vi "FPGA_lock-in_generat-light.vi"() -> ()   [LabVIEW 2010]
uses:
  fast cycles/FPGA_run-states.ctl
  <vilib>/rvi/DataTransferAndStorage/Container/XNode/niFpgaContainer.xnode
  <vilib>/eio/EIONode/EIONode.xnode
  <vilib>/rvi/eio/nirviEIOImplementation/nirviEIOImplementation.xnode
  <vilib>/rvi/eio/common/nirviEmuClasses.ctl
  <vilib>/rvi/FIFO/Fifo_Resource/nirvififoEmulationSetSize.vi
  <vilib>/rvi/DataTransferAndStorage/Container/Common/niFpgaContainerGetUniqueNameForEmu.vi
  <vilib>/rvi/Memory/Memory_Emulation/nirvimemoryEmulationManagerCache_GetValue.vi
  <vilib>/rvi/Memory/Memory_Emulation/nirvimemoryEmulationManagerCache_InsertValue.vi
  <vilib>/Utility/error.llb/Clear Errors.vi
  <vilib>/rvi/Memory/Memory_Emulation/nirvimemoryEmulationManagerCache_SetValue.vi
  <vilib>/rvi/eio/common/nirviEmuTemplateMethod_noerrors.vi
panel:
  in  "DAC mem adr":u8
  out "LI channel":u16
  in  "inhibate lock-in":bool=TRUE
  in  "clock reset":bool
  in  "clock divider":u32=20
  in  "Amplitude":fxp<+/-,16,16>
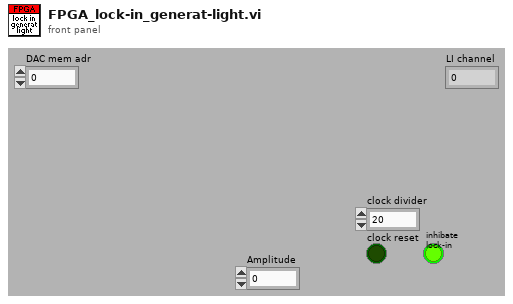
[diagram p1: front panel]
types:
  T1 = typedef "FPGA_run-states.ctl" = enum16{"stopped", "check", "reserve", "run", "release"}
  T2 = cluster{"Boolean array[0]":bool, "Boolean array[1]":bool}
  T3 = typedef "nirviEmuClasses.ctl" = enum16{"IO Read", "IO Write", "Method", "Property Read", "Property Write"}
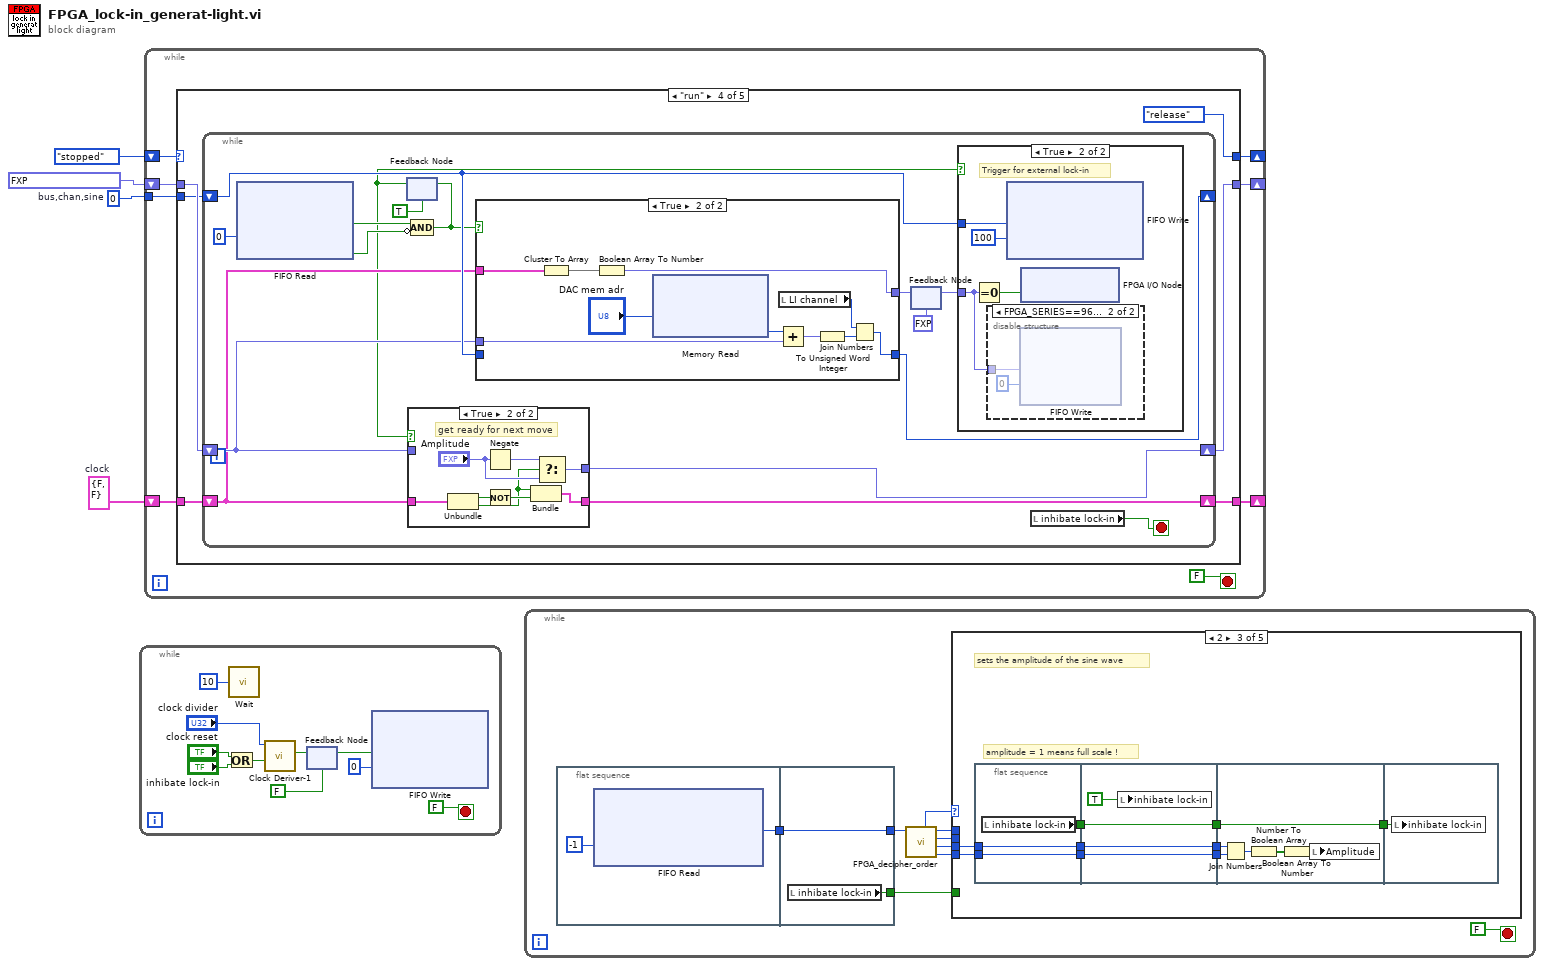
[diagram p0: block diagram]
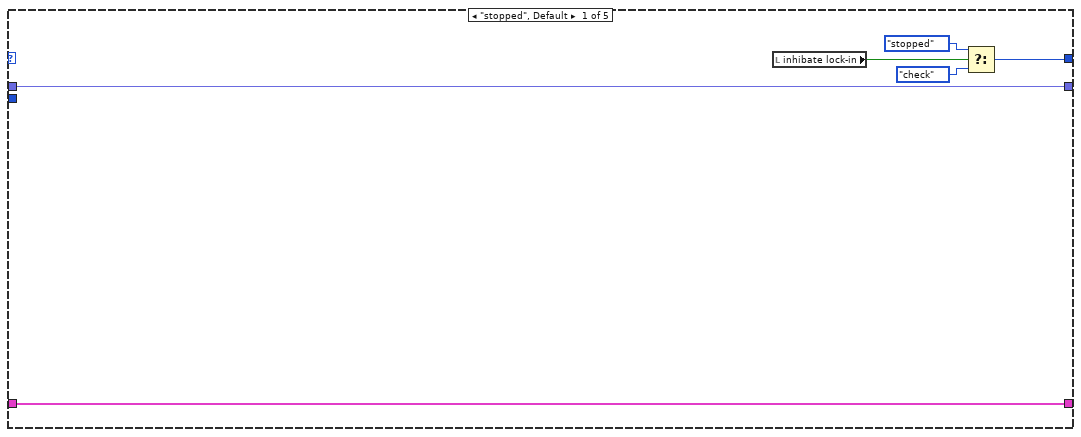
[diagram p2: hidden frame]
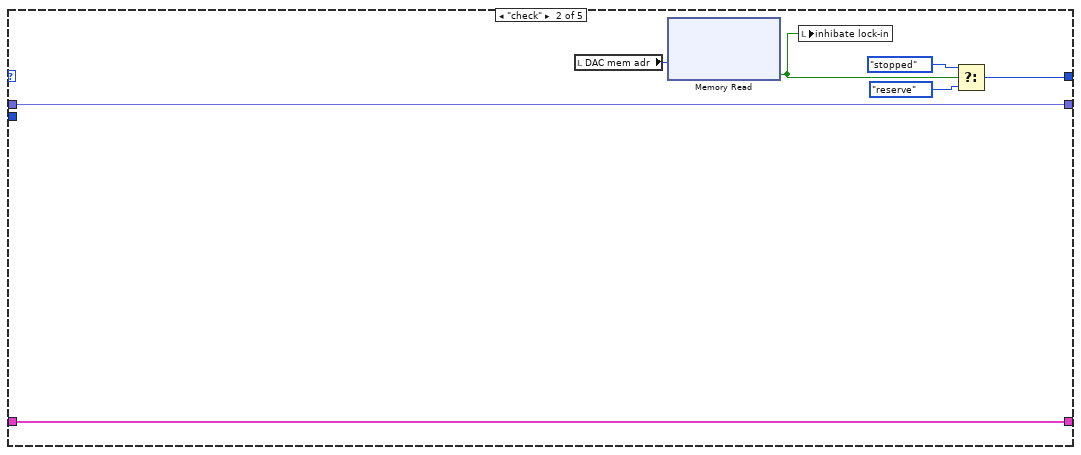
[diagram p3: hidden frame]
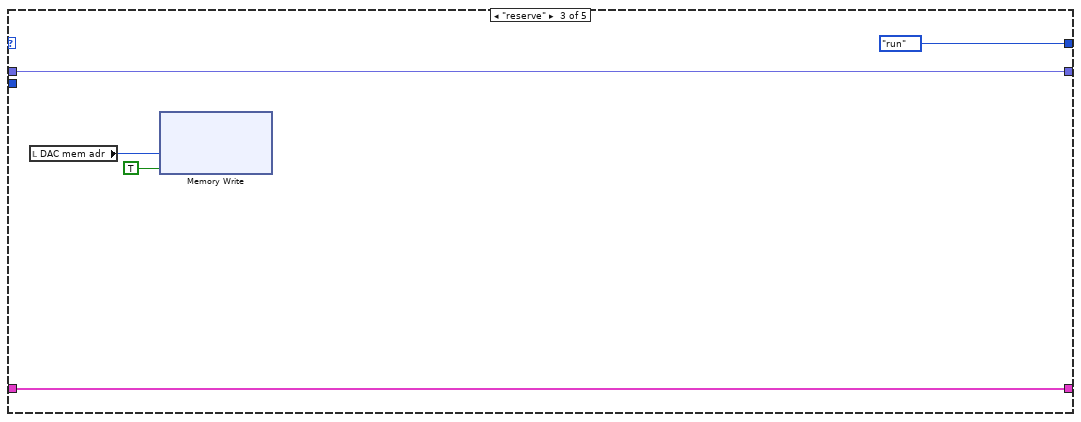
[diagram p4: hidden frame]
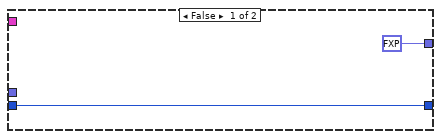
[diagram p8: hidden frame]
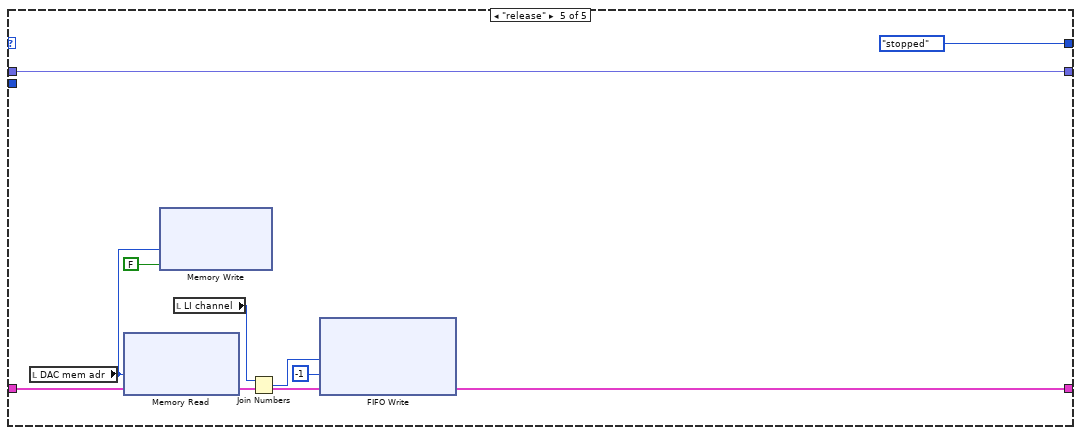
[diagram p9: hidden frame]
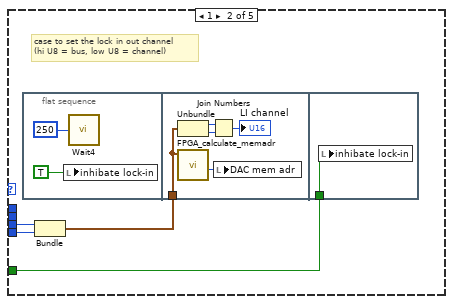
[diagram p11: hidden frame]
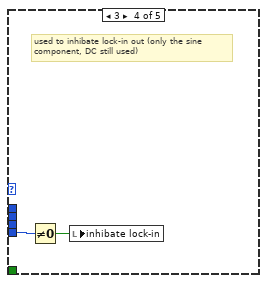
[diagram p12: hidden frame]
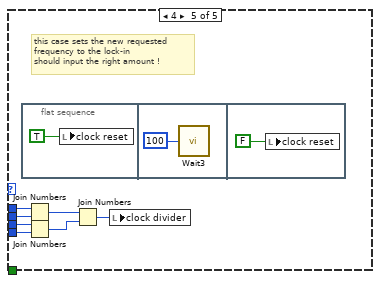
[diagram p13: hidden frame]
diagram:
  w2 = u32 0  # bus,chan,sine
  w3 = T2 {"Boolean array[0]"=FALSE, "Boolean array[1]"=FALSE}  # clock
  n1 = while {
    stop <- FALSE stop-if-true
    n2 = Or(x="clock reset", y="inhibate lock-in") -> (x .or. y?=w11:bool)
    n3 = call "Wait"("Count(uSec)"=u8 10 ("Count(Ticks)")) -> ()  [unwired: 1 out]
    n4 = call "Clock Deriver-1.vi"("Reset"=w11, "Divisor"="clock divider") -> ("Clock Out"=w9:bool)  [unwired: 9 out]
    n5 = feedback-in #1(w9) -> ()
    n6 = feedback #1(FALSE ("Clock Out")) -> (w6:bool)
    n7 = xnode ("FIFO Write")("Element"=w6, "Timeout"=0) -> ()  [unwired: 1 in, 2 out]
  }
  n8 = while {
    shift-right: [w70] -> _
    shift-left: w3 -> [w72]
    shift-right: [w69] -> _
    shift-left: fxp<+/-,16,16> 0.0 ("Amplitude") -> [w73]
    tunnel: w2 -> [w71]
    shift-right: [w67] -> _
    shift-left: FPGA_run-states."stopped" ("run states") -> [w68]
    stop <- FALSE stop-if-true
    n9 = case shown="\"run\"" w68 {
      tunnel: w73 -> [w75 w81 w214 w348 w690]
      tunnel: w72 -> [w74 w82 w213 w347 w689]
      tunnel: w71 -> [_ _ _ w346 _]
      tunnel: [w74 w82 w213 w345 w689] -> w70
      tunnel: [w75 w81 w214 w344 w690] -> w69
      tunnel: [w76 w83 FPGA_run-states."run" ("run states") FPGA_run-states."release" ("run states") FPGA_run-states."stopped" ("run states")] -> w67
      frame "stopped", Default {
        n10 = local read "inhibate lock-in"() -> (w79:bool)
        n11 = Select(t=FPGA_run-states."stopped" ("run states"), s=w79, f=FPGA_run-states."check" ("run states")) -> (s? t:f=w76:T1)
      }
      frame "check" {
        n12 = local read "DAC mem adr"() -> (w86:u8)
        n13 = xnode ("Memory Read")("Address"=w86) -> ("Data"=w80:bool)  [unwired: 1 in, 1 out]
        n14 = local write "inhibate lock-in"(w80) -> ()
        n15 = Select(t=FPGA_run-states."stopped" ("run states"), s=w80, f=FPGA_run-states."reserve" ("run states")) -> (s? t:f=w83:T1)
      }
      frame "reserve" {
        n16 = local read "DAC mem adr"() -> (w217:u8)
        n17 = xnode ("Memory Write")("Address"=w217, "Data"=TRUE) -> ()  [unwired: 1 in, 1 out]
      }
      frame "run" {
        n18 = while {
          shift-right: [w364] -> _
          shift-left: w346 -> [w362]
          shift-right: [w353] -> w345
          shift-left: w347 -> [w352]
          shift-right: [w357] -> w344
          shift-left: w348 -> [w356]
          stop <- w351 stop-if-true
          n19 = xnode ("FIFO Read")("Timeout"=0) -> ("Element"=w361:bool, "Timed Out?"=w359:bool)  [unwired: 1 in, 1 out]
          n20 = feedback #2(TRUE) -> (w349:bool)
          n21 = case shown="True" w349 {
            tunnel: [w417 w425] -> w357
            tunnel: w356 -> [w417 _]
            tunnel: w352 -> [w416 w423]
            tunnel: [w416 w418] -> w353
            frame False {
            }
            frame True {
              # "get ready for next move"
              n22 = Unbundle(w423) -> ("Boolean array[0]"=w421:bool, "Boolean array[1]"=w419:bool)
              n23 = Negate ("Opposé")(x="Amplitude") -> (-x=w424:fxp<+/-,16,16>)
              n24 = Not(x=w421) -> (.not. x?=w420:bool)
              n25 = Bundle("Boolean array[1]"=w419, w420) -> (w418:cluster{"Boolean array[1]":bool, bool})  [unwired: 1 out]
              n26 = Select(t=w424, s=w419, f="Amplitude") -> (s? t:f=w425:fxp<+/-,16,16>)
            }
          }
          n27 = Compound Arithmetic op=AND(w361, invert w359) -> (w350:bool)
          n28 = feedback-in #2(w350) -> ()
          n29 = case shown="True" w350 {
            tunnel: [w546 w553] -> w364
            tunnel: [fxp<+,2,2> 0.0 ("mem adr") w549] -> w363
            tunnel: w362 -> [w546 _]
            tunnel: w356 -> [_ w548]
            tunnel: w352 -> [_ w551]
            frame False {
            }
            frame True {
              n30 = Cluster To Array(cluster=w551) -> (array=w550:bool[])
              n31 = Boolean Array To Number(Boolean array=w550) -> (number=w549:fxp<+,2,2>)
              n32 = xnode ("Memory Read")("Address"="DAC mem adr") -> ("Data"=w547:u16)  [unwired: 1 in, 1 out]
              n33 = Add(x=w547, y=w548) -> (x+y=w556:fxp<+,16,16>)
              n34 = local read "LI channel"() -> (w555:u16)
              n35 = To Unsigned Word Integer(number=w556) -> (unsigned 16bit integer=w554:u16)
              n36 = Join Numbers(hi=w555, lo=w554) -> ((hi.lo)=w553:u32)
            }
          }
          n37 = feedback-in #3(w363) -> ()
          n38 = feedback #3(fxp<+,2,2> 0.0 ("mem adr")) -> (w355:fxp<+,2,2>)
          n39 = case shown="True" w349 {
            tunnel: w362 -> [_ w428]
            tunnel: w355 -> [_ w426]
            frame False {
            }
            frame True {
              # "Trigger for external lock-in"
              n40 = Equal To 0?(x=w426) -> (x = 0?=w427:bool)
              n41 = disable-structure shown="FPGA_SERIES==9612" {
                disable-tunnel: w426 -> [_ w482]
                frame condition #0 (active) {
                }
                frame condition #1 {
                  n42 = xnode ("FIFO Write")("Element"=w482, "Timeout"=0) -> ()  [unwired: 1 in, 2 out]
                }
              }
              n43 = xnode ("FIFO Write")("Element"=w428, "Timeout"=100) -> ()  [unwired: 1 in, 2 out]
              n44 = xnode "FPGA I/O Node"("Port9/DIO0"=w427) -> ()  [unwired: 1 in, 1 out]
            }
          }
          n45 = local read "inhibate lock-in"() -> (w351:bool)
        }
      }
      frame "release" {
        n46 = local read "DAC mem adr"() -> (w687:u8)
        n47 = xnode ("Memory Read")("Address"=w687) -> ("Data"=w685:u16)  [unwired: 1 in, 1 out]
        n48 = xnode ("Memory Write")("Address"=w687, "Data"=FALSE) -> ()  [unwired: 1 in, 1 out]
        n49 = local read "LI channel"() -> (w688:u16)
        n50 = Join Numbers(hi=w688, lo=w685) -> ((hi.lo)=w684:u32)
        n51 = xnode ("FIFO Write")("Element"=w684, "Timeout"=-1) -> ()  [unwired: 1 in, 2 out]
      }
    }
  }
  n52 = while {
    stop <- FALSE stop-if-true
    n53 = flat-sequence {
      tunnel: [w1003] -> w995
      tunnel: [w1057] -> w1001
      tunnel: w995 -> [w1057]
      tunnel: [w1056] -> w994
      frame #0 {
        n54 = xnode ("FIFO Read")("Timeout"=-1) -> ("Element"=w1003:u64)  [unwired: 1 in, 2 out]
      }
      frame #1 {
        n55 = local read "inhibate lock-in"() -> (w1056:bool)
      }
    }
    n56 = call "FPGA_decipher_order.vi"("order in"=w1001) -> ("data 1"=w999:u8, "data 2"=w998:u8, "data 3"=w997:u8, "data 4"=w996:u8, "order out"=w1000:u8)  [unwired: 6 out]
    n57 = case shown="2" w1000 {
      tunnel: w999 -> [_ w1060 w1077 w1094 w1098]
      tunnel: w998 -> [_ w1061 w1078 _ w1099]
      tunnel: w997 -> [_ _ _ _ w1100]
      tunnel: w996 -> [_ _ _ _ w1101]
      tunnel: w994 -> [_ w1058 _ _ _]
      frame 0, Default {
      }
      frame 1 {
        # "case to set the lock in out channel\n(hi U8 = bus, low U8 = channel)"
        n58 = flat-sequence {
          tunnel: w1059 -> [w1067]
          tunnel: w1058 -> [w1069]
          frame #0 {
            n59 = local write "inhibate lock-in"(TRUE ("inhibate lock-in")) -> ()
            n60 = call "Wait4"("Count(uSec)"=u8 250) -> ()  [unwired: 1 out]
          }
          frame #1 {
            n61 = Unbundle(w1067) -> ("data 2"=w1065:u8, "data 1"=w1066:u8)
            n62 = call "FPGA_calculate_memadr.vi"("Cluster"=w1067) -> ("mem adr"=w1068:u8)  [unwired: 10 out]
            n63 = Join Numbers(hi=w1065, lo=w1066) -> ((hi.lo)=→"LI channel":u16)
            n64 = local write "DAC mem adr"(w1068) -> ()
          }
          frame #2 {
            n65 = local write "inhibate lock-in"(w1069) -> ()
          }
        }
        n66 = Bundle("data 2"=w1061, "data 1"=w1060) -> (w1059:cluster{"data 2":u8, "data 1":u8})  [unwired: 1 out]
      }
      frame 2 {
        # "amplitude = 1 means full scale !"
        # "sets the amplitude of the sine wave"
        n67 = flat-sequence {
          tunnel: w1078 -> [w1079]
          tunnel: w1077 -> [w1080]
          tunnel: [w1081] -> w1074
          tunnel: [w1080] -> w1073
          tunnel: [w1079] -> w1070
          tunnel: [w1084] -> w1075
          tunnel: w1074 -> [w1084]
          tunnel: w1073 -> [w1083]
          tunnel: [w1083] -> w1072
          tunnel: [w1082] -> w1071
          tunnel: w1070 -> [w1082]
          tunnel: [w1091] -> w1076
          tunnel: w1075 -> [w1091]
          tunnel: w1072 -> [w1087]
          tunnel: w1071 -> [w1086]
          tunnel: w1076 -> [w1092]
          frame #0 {
            n68 = local read "inhibate lock-in"() -> (w1081:bool)
          }
          frame #1 {
            n69 = local write "inhibate lock-in"(TRUE ("inhibate lock-in")) -> ()
          }
          frame #2 {
            n70 = Join Numbers(hi=w1086, lo=w1087) -> ((hi.lo)=w1090:u16)
            n71 = Number To Boolean Array(number=w1090) -> (Boolean array=w1088:bool[])
            n72 = Boolean Array To Number(Boolean array=w1088) -> (number=w1089:fxp<+/-,16,16>)
            n73 = local write "Amplitude"(w1089) -> ()
          }
          frame #3 {
            n74 = local write "inhibate lock-in"(w1092) -> ()
          }
        }
      }
      frame 3 {
        # "used to inhibate lock-in out (only the sine\ncomponent, DC still used)"
        n75 = Not Equal To 0?(x=w1094) -> (x != 0?=w1093:bool)
        n76 = local write "inhibate lock-in"(w1093) -> ()
      }
      frame 4 {
        # "this case sets the new requested\nfrequency to the lock-in\nshould input the right amount !"
        n77 = flat-sequence {
          frame #0 {
            n78 = local write "clock reset"(TRUE ("clock reset")) -> ()
          }
          frame #1 {
            n79 = call "Wait3"("Count(uSec)"=u8 100) -> ()  [unwired: 1 out]
          }
          frame #2 {
            n80 = local write "clock reset"(FALSE ("clock reset")) -> ()
          }
        }
        n81 = Join Numbers(hi=w1101, lo=w1100) -> ((hi.lo)=w1097:u16)
        n82 = Join Numbers(hi=w1099, lo=w1098) -> ((hi.lo)=w1096:u16)
        n83 = Join Numbers(hi=w1097, lo=w1096) -> ((hi.lo)=w1095:u32)
        n84 = local write "clock divider"(w1095) -> ()
      }
    }
  }
